vi "Read IQ TDMS File.vi"(8 "error in (no error)":errorcluster, 11 "tdms ref in":refnum<k34>) -> (0 "error out":errorcluster, 2 "wfm array":waveform(cdb)[](array[waveform]), 3 "tdms ref out":refnum<k34>)   [LabVIEW 2021]
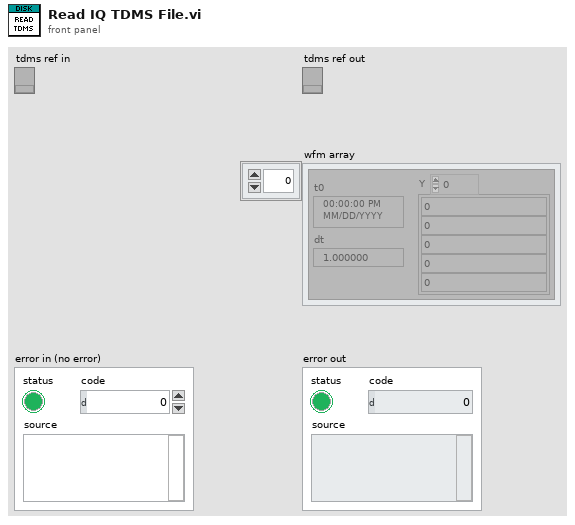
[diagram p1: front panel]
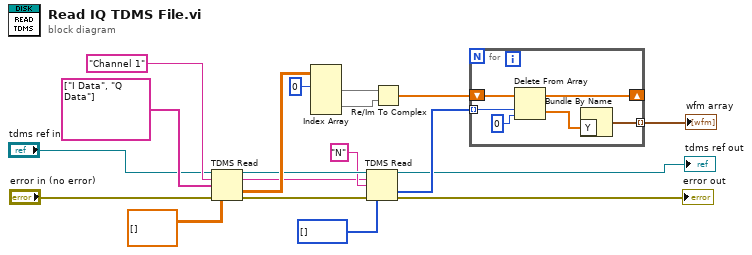
[diagram p0: block diagram]
diagram:
  n1 = TDMS Read(0:"tdms ref in", 5:"Channel 1" ("group name in"), 7:string[] ["I Data", "Q Data"] ("group name in"), 11:"error in (no error)", 12:dbl[][] []) -> (4:w11:refnum<k34>, 6:w8:string, 10:w12:dbl[][], 15:w7:errorcluster)  [unwired: 3 in, 2 out]
  n2 = Index Array(array=w12, index (row) #1=0 ("disabled index (col)")) -> (element #1=w13:dbl[], element #2=w14:dbl[])  [unwired: 3 in]
  n3 = TDMS Read(0:w11, 5:w8, 7:"N" ("channel name(s) in"), 11:w7, 12:i32[] []) -> (4:→"tdms ref out":refnum<k34>, 10:w18:i32[], 15:→"error out":errorcluster)  [unwired: 3 in, 3 out]
  n4 = Re/Im To Complex(1:w14, 2:w13) -> (0:w15:cdb[])
  n5 = for {
    tunnel: w18 -> [w24] mode=indexing
    shift-right: [w20] -> _
    shift-left: w15 -> [w25]
    tunnel: [w21] -> w19 mode=indexing
    n6 = Delete From Array(array=w25, length=w24, index=0) -> (deleted portion=w22:cdb[], array with subset deleted=w20:cdb[])
    n7 = Bundle By Name("Y"=w22) -> (w21:waveform(cdb))  [unwired: 1 in]
  }
  "wfm array" <- w19
